vi "test Find and Initialize SLSC Switch CD.vi"(8 "error in (no error)":errorcluster, 11 "TestCase in":refnum<class "SLSC Switch Scripting Unit Tests.lvclass">) -> (0 "error out":errorcluster, 3 "TestCase out":refnum<class "SLSC Switch Scripting Unit Tests.lvclass">)   [LabVIEW 2017, in "SLSC Switch Scripting Unit Tests.lvclass"]
uses:
  SLSC Switch Scripting Unit Tests.lvclass
  <vilib>/NI Veristand/Custom Device API/Custom Device Item Ref.ctl
  SLSC Switch Scripting Unit Tests.lvclass/SLSC Switch Scripting Unit Tests.ctl
  Custom Device/Find All SLSC Switch Custom Devices.vi
  Custom Device/Find SLSC Switch Custom Device by Name.vi
  <vilib>/addons/_JKI Toolkits/VI Tester/TestCase.llb/TestCase.lvclass
  SLSC Switch Scripting.lvlib
  <vilib>/NI VeriStand/Custom Device API/Custom Device API.lvlib
  C:/Program Files (x86)/National Instruments/LabVIEW 2017/vi.lib/addons/_JKI Toolkits/VI Tester/TestCase.llb/TestCase.lvclass
panel:
  in  "Save?":bool
  out "Output Filename":string
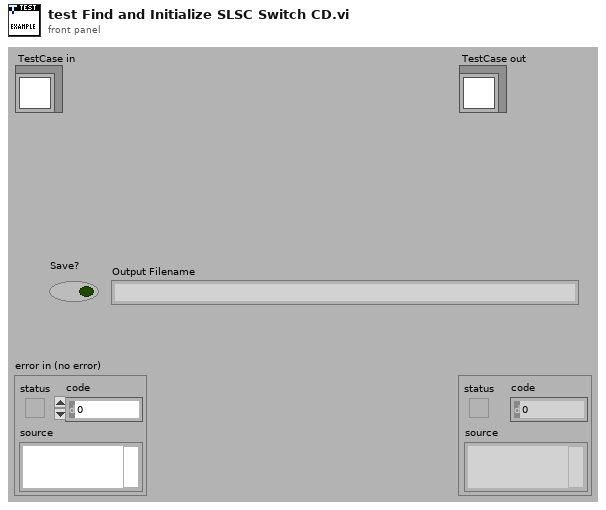
[diagram p1: front panel]
types:
  T1 = typedef "Custom Device API.lvlib/Custom Device Item Ref.ctl" = u64
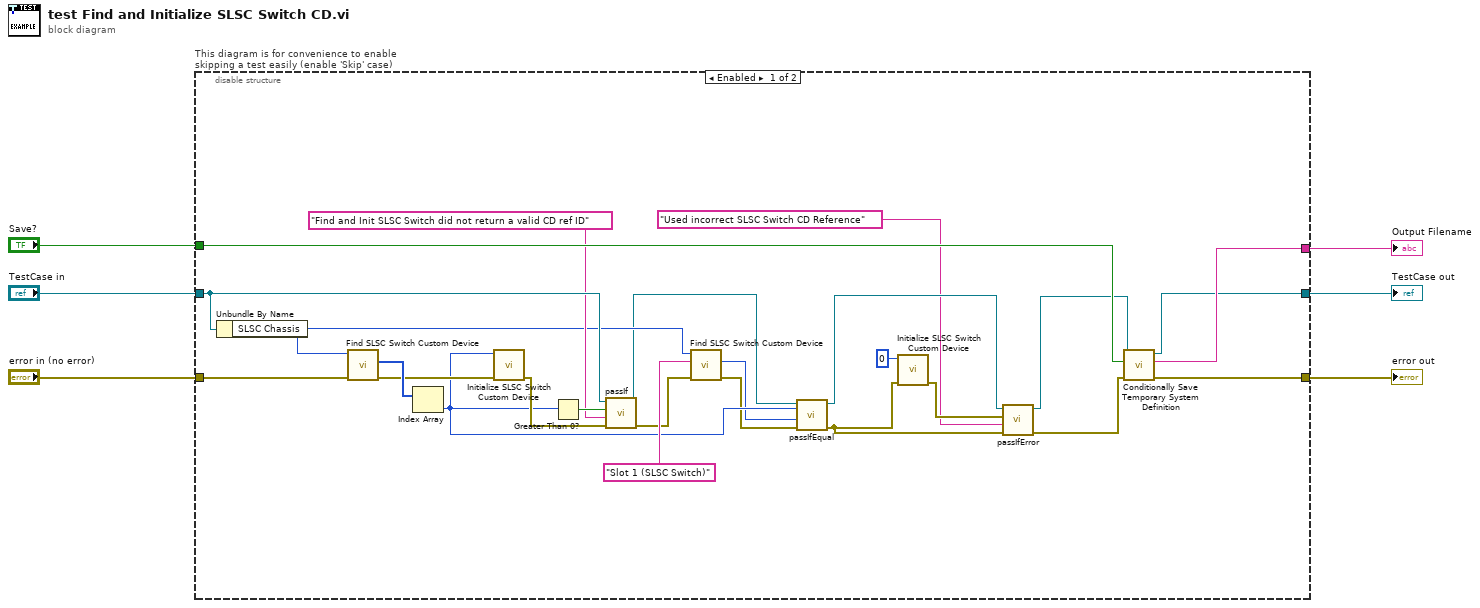
[diagram p0: block diagram]
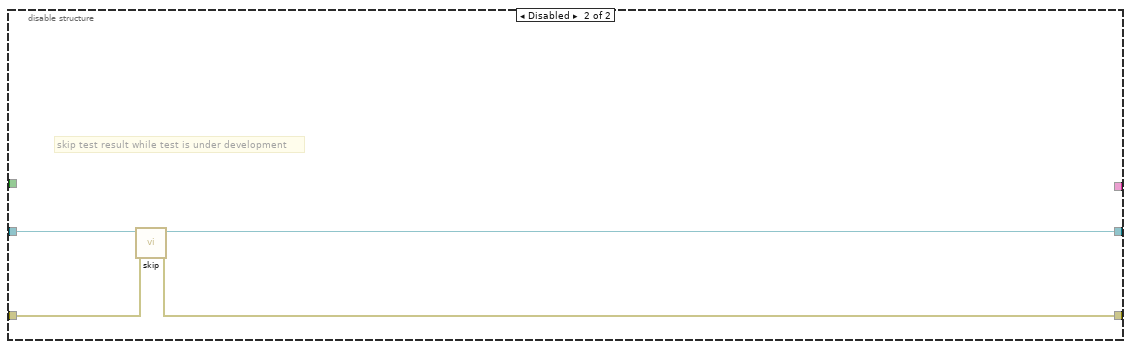
[diagram p2: hidden frame]
diagram:
  n1 = disable-structure "This diagram is for convenience to enable skipping a test easily (enable 'Skip' case)" shown="Enabled" {
    disable-tunnel: "TestCase in" -> [w27 w35]
    disable-tunnel: [w29 w33] -> w3
    disable-tunnel: [w30 w34] -> w5
    disable-tunnel: "error in (no error)" -> [w22 w32]
    disable-tunnel: [w31 _] -> w2
    disable-tunnel: "Save?" -> [w26 _]
    frame Enabled {
      n2 = Unbundle By Name(w27) -> ("SLSC Chassis"=w20:u64)
      n3 = call-poly "Find SLSC Switch Custom Device.vi"("error in (no error)"=w22, "SLSC Chassis Ref"=w20) -> ("error out"=w23:errorcluster, "SLSC Switch Custom Device Ref IDs"=w24:T1[])  [unwired: 7 in, 1 out]
      n4 = Index Array(array=w24) -> (element=w18:T1)  [unwired: 1 in]
      n5 = call "Initialize SLSC Switch Custom Device.vi"("error in (no error)"=w23, "SLSC Switch Custom Device Ref in"=w18) -> ("error out"=w21:errorcluster)  [unwired: 7 in, 2 out]
      n6 = Greater Than 0?(x=w18) -> (x > 0?=w28:bool)
      n7 = call-dynamic "passIf.vi"("error in (no error)"=w21, "message (\"\")"="Find and Init SLSC Switch did not return a valid CD ref ID" ("message (\"\")"), "pass"=w28, "TestCase in"=w27) -> ("error out"=w15:errorcluster, "TestCase out"=w16:refnum<class "SLSC Switch Scripting Unit Tests.lvclass">)  [unwired: 6 in]
      n8 = call-poly "Find SLSC Switch Custom Device.vi"("error in (no error)"=w15, "Name"="Slot 1 (SLSC Switch)", "SLSC Chassis Ref"=w20) -> ("error out"=w14:errorcluster, "SLSC Switch Custom Device Ref"=w17:T1)  [unwired: 6 in, 1 out]
      n9 = call-dynamic "passIfEqual.vi"("error in (no error)"=w14, "y"=w17, "x"=w18, "TestCase in"=w16) -> ("error out"=w9:errorcluster, "TestCase out"=w12:refnum<class "SLSC Switch Scripting Unit Tests.lvclass">)  [unwired: 6 in]
      n10 = call "Initialize SLSC Switch Custom Device.vi"("error in (no error)"=w9, "SLSC Switch Custom Device Ref in"=T1 0) -> ("error out"=w13:errorcluster)  [unwired: 7 in, 2 out]
      n11 = call-dynamic "passIfError.vi"("error in (no error)"=w9, "task (\"\")"="Used incorrect SLSC Switch CD Reference" ("task (\"\")"), "error"=w13, "TestCase in"=w12) -> ("error out"=w8:errorcluster, "TestCase out"=w11:refnum<class "SLSC Switch Scripting Unit Tests.lvclass">)  [unwired: 6 in]
      n12 = call "Conditionally Save Temporary System Definition.vi"("error in (no error)"=w8, "Save?"=w26, "Test Case"=w11) -> ("error out"=w30:errorcluster, "filename"=w31:string, "Test Case"=w29:refnum<class "SLSC Switch Scripting Unit Tests.lvclass">)  [unwired: 6 in]
    }
    frame Disabled {
      # "skip test result while test is under development"
      n13 = call <vilib>:"skip.vi"("error in (no error)"=w32, "TestCase in"=w35) -> ("error out"=w34:errorcluster, "TestCase out"=w33:refnum<class "SLSC Switch Scripting Unit Tests.lvclass">)  [unwired: 8 in]
    }
  }
  "error out" <- w5
  "TestCase out" <- w3
  "Output Filename" <- w2
